vi "StartUp.vi"(8 "error in (no error)":errorcluster, 11 "AppLogger in":refnum<class "AppLogger.lvclass">) -> (0 "error out":errorcluster, 3 "AppLogger out":refnum<class "AppLogger.lvclass">)   [LabVIEW 2014, in "AppLogger.lvclass"]
uses:
  AppLogger.lvclass
  Process Loop.vi
panel:
  in  "Filename":string
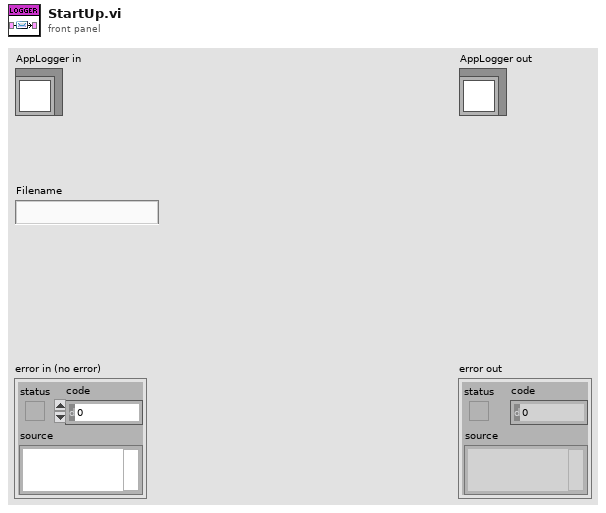
[diagram p1: front panel]
types:
  T1 = enum16{"open", "replace", "create", "open or create", "replace or create", "replace or create with confirmation"}
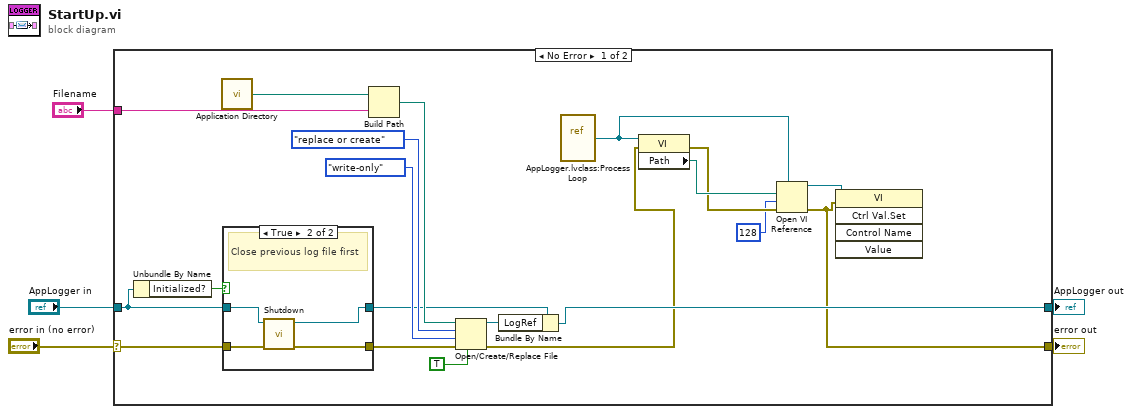
[diagram p0: block diagram]
diagram:
  n1 = case shown="No Error" "error in (no error)" {
    selector: "error in (no error)" -> [w16 w33]
    tunnel: [w6 w33] -> w4
    tunnel: [w19 w32] -> w2
    tunnel: "AppLogger in" -> [w14 w32]
    tunnel: "Filename" -> [w24 _]
    frame No Error {
      n2 = Unbundle By Name(w14) -> ("Initialized?"=w17:bool)
      n3 = call <vilib>:"Application Directory.vi"() -> ("Application Directory"=w25:path)
      n4 = case shown="True" w17 {
        tunnel: w14 -> [w27 w31]
        tunnel: w16 -> [w26 w30]
        tunnel: [w26 w29] -> w15
        tunnel: [w27 w28] -> w13
        frame False {
          # "We're ok to start up"
        }
        frame True {
          # "Close previous log file first"
          n5 = call "Shutdown.vi"("error in (no error)"=w30, "AppLogger in"=w31) -> ("error out"=w29:errorcluster, "AppLogger out"=w28:refnum<class "AppLogger.lvclass">)  [unwired: 8 in]
        }
      }
      n6 = Build Path(base path=w25, name or relative path=w24) -> (appended path=w23:path)
      n7 = Open/Create/Replace File(file path (use dialog)=w23, error in=w15, operation (0:open)=T1."replace or create", access (0:read/write)=enum16{"read/write", "read-only", "write-only"}."write-only", disable buffering (F)=TRUE) -> (refnum out=w18:refnum<file>, error out=w11:errorcluster)  [unwired: 1 in, 1 out]
      n8 = Bundle By Name(cluster=w13, "LogRef"=w18) -> (w19:refnum<class "AppLogger.lvclass">)
      n9 = vi-ref "AppLogger.lvclass:Process Loop.vi"() -> (w9:refnum<vi>)
      n10 = property class="VI"(reference=w9, error in=w11) -> (error out=w10:errorcluster, "Path"=w12:path)  [unwired: 1 out]
      n11 = Open VI Reference(type specifier VI Refnum (for type only)=w9, vi path=w12, options=128, error in (no error)=w10) -> (vi reference=w7:refnum<vi>, error out=w6:errorcluster)  [unwired: 2 in]
      n12 = invoke class="VI" method="Ctrl Val.Set"(reference=w7, error in=w6) -> ()  [unwired: 3 in, 5 out]
    }
    frame Error {
    }
  }
  "error out" <- w4
  "AppLogger out" <- w2
